vi "update_sampling_mode.vi"(8 "error in (no error)":errorcluster, 11 "DAQmxWriteSignals in":refnum<class "SignalWriterMM140725DAQmx.lvclass">) -> (0 "error out":errorcluster, 3 "DAQmxWriteSignals out":refnum<class "SignalWriterMM140725DAQmx.lvclass">)   [LabVIEW 2010, in "SignalWriterMM140725DAQmx.lvclass"]
uses:
  SignalWriterMM140725DAQmx.lvclass
  <vilib>/DAQmx/configure/timing.llb/DAQmx Timing (Sample Clock).vi
  <vilib>/DAQmx/configure/trigger.llb/DAQmx Start Trigger (None).vi
  <vilib>/DAQmx/configure/trigger.llb/DAQmx Start Trigger (Digital Edge).vi
  Program Files (x86)/National Instruments/LabVIEW 2010/resource/objmgr/daqmx.rc
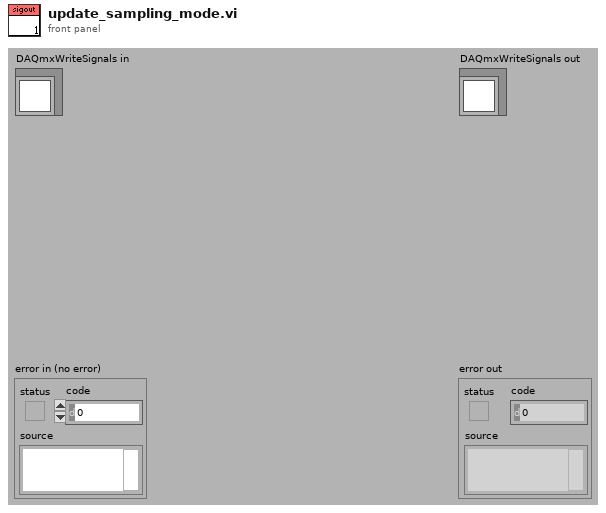
[diagram p1: front panel]
types:
  T1 = typedef "SignalWriterMM140725DAQmx.lvclass/trigger_edge_enum.ctl" = enum16{"rising", "falling"}
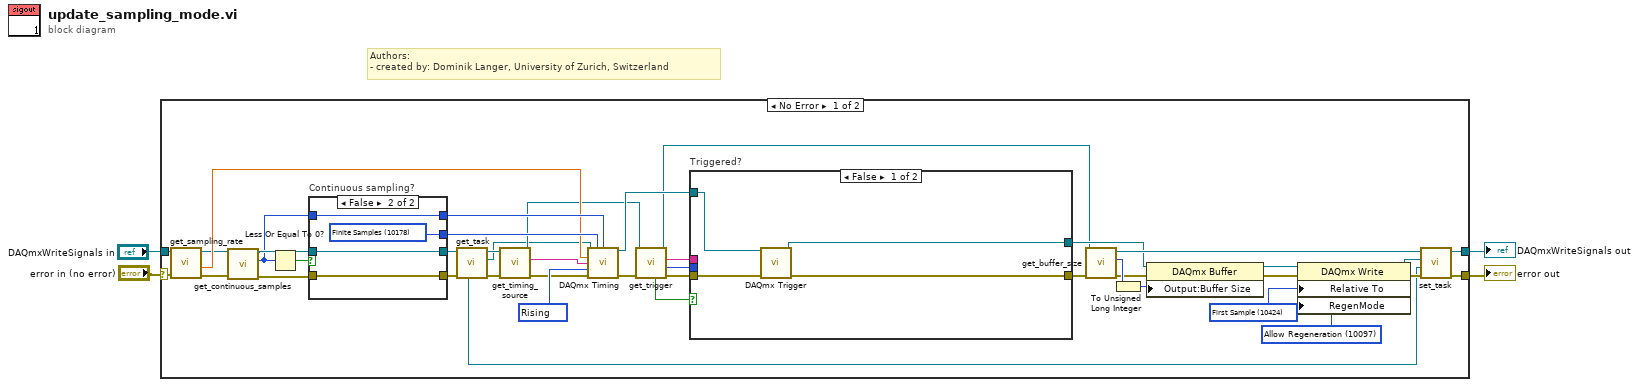
[diagram p0: block diagram]
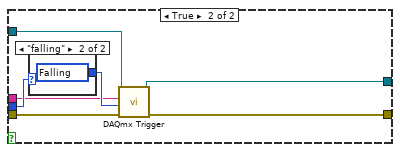
[diagram p2: hidden frame]
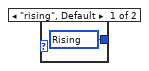
[diagram p3: hidden frame]
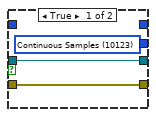
[diagram p4: hidden frame]
diagram:
  # "Authors: \n- created by: Dominik Langer, University of Zurich, Switzerland"
  n1 = case shown="No Error" "error in (no error)" {
    selector: "error in (no error)" -> [w26 w68]
    tunnel: [w18 w68] -> w3
    tunnel: [w17 w67] -> w2
    tunnel: "DAQmxWriteSignals in" -> [w25 w67]
    frame No Error {
      w44 = 10280 items=["Rising"=10280, "Falling"=10171] ("active edge")
      w35 = 10097 items=["Allow Regeneration"=10097, "Do Not Allow Regeneration"=10158] ("RegenMode")
      w27 = 10424 items=["First Sample"=10424, "Current Write Position"=10430] ("RelativeTo")
      n2 = call-dynamic "get_sampling_rate.vi"("error in (no error)"=w26, "GenericWriteSignals in"=w25) -> ("error out"=w37:errorcluster, "sampling rate (Hz)"=w39:dbl, "GenericWriteSignals out"=w38:refnum<class "SignalWriterMM140725DAQmx.lvclass">)  [unwired: 7 out]
      n3 = call-dynamic "get_continuous_samples.vi"("error in (no error)"=w37, "GenericWriteSignals.lvclass in"=w38) -> ("error out"=w46:errorcluster, "continuous samples"=w19:i32, "GenericWriteSignals.lvclass out"=w45:refnum<class "SignalWriterMM140725DAQmx.lvclass">)  [unwired: 7 out]
      n4 = Less Or Equal To 0?(x=w19) -> (x <= 0?=w20:bool)
      n5 = case "Continuous sampling?" shown="False" w20 {
        tunnel: [w61 w65] -> w24
        tunnel: [w60 w64] -> w23
        tunnel: w46 -> [w61 w65]
        tunnel: w45 -> [w60 w64]
        tunnel: [w62 w66] -> w42
        tunnel: [_ w63] -> w43
        tunnel: w19 -> [_ w63]
        frame True {
          w62 = 10123 items=["Finite Samples"=10178, "Continuous Samples"=10123, "Hardware Timed Single Point"=12522] ("sample mode")
        }
        frame False {
          w66 = 10178 items=["Finite Samples"=10178, "Continuous Samples"=10123, "Hardware Timed Single Point"=12522] ("sample mode")
        }
      }
      n6 = call-dynamic "get_task.vi"("error in (no error)"=w24, "DAQmxWriteSignals in"=w23) -> ("error out"=w21:errorcluster, "writer task"=w6:refnum<k21>, "DAQmxWriteSignals out"=w22:refnum<class "SignalWriterMM140725DAQmx.lvclass">, "counter task"=w5:refnum<k21>)  [unwired: 6 out]
      n7 = call-dynamic "get_timing_source.vi"("error in (no error)"=w21, "DAQmxWriteSignals.lvclass in"=w22) -> ("error out"=w41:errorcluster, "timing source"=w40:tag, "DAQmxWriteSignals.lvclass out"=w10:refnum<class "SignalWriterMM140725DAQmx.lvclass">)  [unwired: 7 out]
      n8 = call-poly <vilib>:"DAQmx Timing.vi"("task/channels in"=w6, "sample mode"=w42, "samples per channel"=w43, "rate"=w39, "source"=w40, "active edge"=w44, "error in"=w41) -> ("task out"=w16:refnum<k21>, "error out"=w13:errorcluster)  [unwired: 7 out]
      n9 = call-dynamic "get_trigger.vi"("error in (no error)"=w13, "DAQmxWriteSignals in"=w10) -> ("error out"=w12:errorcluster, "edge"=w9:T1, "digital trigger line"=w8:tag, "DAQmxWriteSignals out"=w7:refnum<class "SignalWriterMM140725DAQmx.lvclass">, "trigger set?"=w11:bool)  [unwired: 5 out]
      n10 = case "Triggered?" shown="False" w11 {
        tunnel: w16 -> [w47 w57]
        tunnel: [w48 w51] -> w15
        tunnel: w12 -> [w50 w56]
        tunnel: [w49 w52] -> w14
        tunnel: w9 -> [_ w54]
        tunnel: w8 -> [_ w53]
        frame False {
          n11 = call-poly <vilib>:"DAQmx Trigger.vi"("task/channels in"=w47, "error in"=w50) -> ("task out"=w48:refnum<k21>, "error out"=w49:errorcluster)  [unwired: 12 out]
        }
        frame True {
          n12 = case shown="\"falling\"" w54 {
            tunnel: [w58 w59] -> w55
            frame "rising", Default {
              w58 = 10280 items=["Rising"=10280, "Falling"=10171] ("edge")
            }
            frame "falling" {
              w59 = 10171 items=["Rising"=10280, "Falling"=10171] ("edge")
            }
          }
          n13 = call-poly <vilib>:"DAQmx Trigger.vi"("task/channels in"=w57, "source"=w53, "edge"=w55, "error in"=w56) -> ("task out"=w51:refnum<k21>, "error out"=w52:errorcluster)  [unwired: 10 out]
        }
      }
      n14 = call-dynamic "get_buffer_size.vi"("error in (no error)"=w14, "GenericWriteSignals.lvclass in"=w7) -> ("error out"=w31:errorcluster, "buffer size (samples)"=w33:i32, "GenericWriteSignals.lvclass out"=w32:refnum<class "SignalWriterMM140725DAQmx.lvclass">)  [unwired: 7 out]
      n15 = To Unsigned Long Integer(number=w33) -> (unsigned 32bit integer=w34:u32)
      n16 = property class="DAQmx Buffer"(reference=w15, error in=w31, "Output:Buffer Size"=w34) -> (reference out=w36:refnum<k21>, error out=w28:errorcluster)
      n17 = property class="DAQmx Write"(reference=w36, error in=w28, "Relative To"=w27, "RegenMode"=w35) -> (reference out=w30:refnum<k21>, error out=w29:errorcluster)
      n18 = call-dynamic "set_task.vi"("error in (no error)"=w29, "counter task"=w5, "output task"=w30, "DAQmxWriteSignals in"=w32) -> ("error out"=w18:errorcluster, "DAQmxWriteSignals out"=w17:refnum<class "SignalWriterMM140725DAQmx.lvclass">)  [unwired: 6 out]
    }
    frame Error {
    }
  }
  "error out" <- w3
  "DAQmxWriteSignals out" <- w2
